vi "Write Error Log Entry.vi"(7 "Classification":T1, 8 "error in (no error)":errorcluster, 9 "current time":timestamp, 10 "Account #":u32, 11 "Log Ref In":refnum<file>) -> (0 "error out":errorcluster, 3 "Log Ref Out":refnum<file>)   [LabVIEW 2012]
uses:
  TypeDefs/Error Classification.ctl
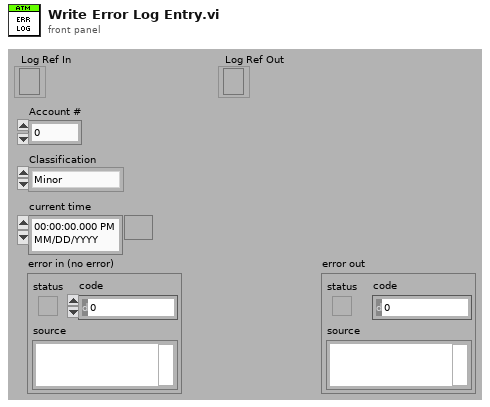
[diagram p1: front panel]
types:
  T1 = typedef "Error Classification.ctl" = enum16{"Minor", "Session", "System"}
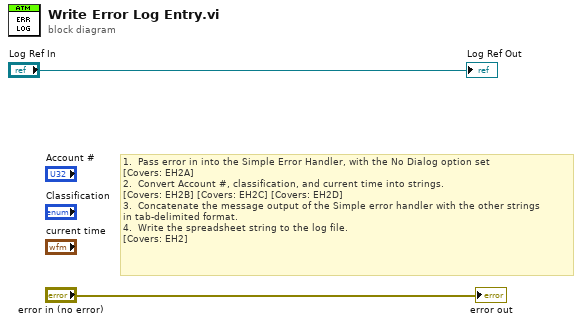
[diagram p0: block diagram]
diagram:
  # "1.  Pass error in into the Simple Error Handler, with the No Dialog option set\n[Covers: EH2A]\n2.  Convert Account #, classification, and current time into strings.\n[Covers: EH2B] [Covers: EH2C] [Covers: EH2D]\n3.  Concatenate the message output of the Simple error handler with the other strings\nin tab-delimited format.\n4.  Write the spreadsheet string to the log file.\n[Covers: EH2]"
  "Log Ref Out" <- "Log Ref In"
  "error out" <- "error in (no error)"
